vi "GlobalGetMesaurementStatus.vi"() -> ()   [LabVIEW 2011]
panel:
  out "FifoMesaurementTerminatior":bool
  out "MeasurementAktiv":bool
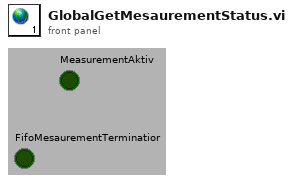
[diagram p1: front panel]
diagram:
